vi "Ejercicio_14_Adquisicion_Datos_DAQ.vi"() -> ()   [LabVIEW 2021]
panel:
  out "Waveform Chart":dbl(graph)
  in  "stop":bool
  out "Boolean":bool
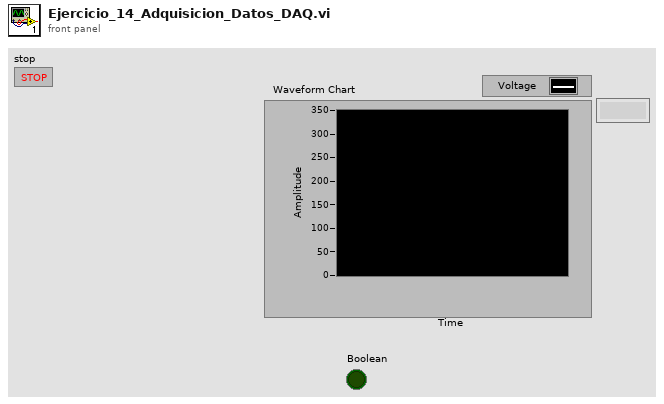
[diagram p1: front panel]
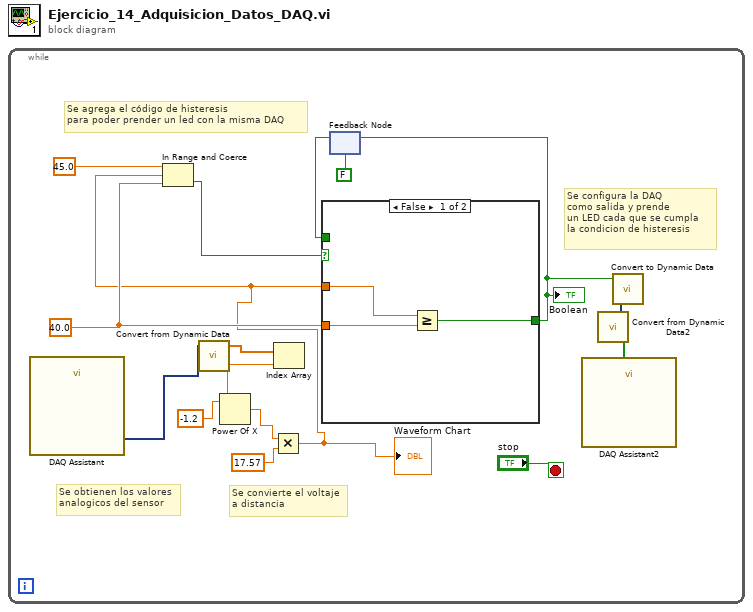
[diagram p0: block diagram]
diagram:
  n1 = while {
    stop <- "stop" stop-if-true
    w12 = 40.0 ("lower limit")
    # "Se configura la DAQ\ncomo salida y prende\nun LED cada que se cumpla \nla condicion de histeresis"
    # "Se agrega el código de histeresis\npara poder prender un led con la misma DAQ"
    # "Se convierte el voltaje\na distancia"
    # "Se obtienen los valores\nanalogicos del sensor"
    n2 = call "DAQ Assistant"() -> ("data"=w9:dynamicdata)  [unwired: 17 in, 2 out]
    n3 = call "Convert from Dynamic Data"("Dynamic Data Type"=w9) -> ("Array"=w8:dbl[])  [unwired: 3 in]
    n4 = Index Array(array=w8) -> (element=w6:dbl)  [unwired: 1 in]
    n5 = Power Of X(1:w6, 2:-1.2 ("y")) -> (0:w5:dbl)
    n6 = Multiply(x=w5, y=17.57) -> (x*y=w4:dbl)
    "Waveform Chart" <- w4
    n7 = In Range and Coerce(upper limit=45.0, x=w4, lower limit=w12) -> (In Range?=w15:bool)  [unwired: 1 out]
    n8 = feedback #1(FALSE) -> (w14:bool)
    n9 = case shown="False" w15 {
      tunnel: w14 -> [_ w20]
      tunnel: w4 -> [w19 _]
      tunnel: w12 -> [w18 _]
      tunnel: [w17 w20] -> w3
      frame False {
        n10 = Greater Or Equal?(x=w19, y=w18) -> (x >= y?=w17:bool)
      }
      frame True {
      }
    }
    "Boolean" <- w3
    n11 = feedback-in #1(w3) -> ()
    n12 = call "Convert to Dynamic Data"("Boolean"=w3) -> ("Dynamic Data Type"=w2:dynamicdata)  [unwired: 3 in]
    n13 = call "Convert from Dynamic Data2"("Dynamic Data Type"=w2) -> ("Array"=w1:bool[])  [unwired: 3 in]
    n14 = call "DAQ Assistant2"("data"=w1) -> ()  [unwired: 17 in, 2 out]
  }
